vi "Ex2.vi"   [LabVIEW 2012]
uses:
  <userlib>/rosforlv/ROS/Code/SubVIs/BaxterSide.ctl
panel:
  # "Hit run to close and open the gripper"
types:
  T1 = typedef "BaxterSide.ctl" = enum16{"left", "right"}
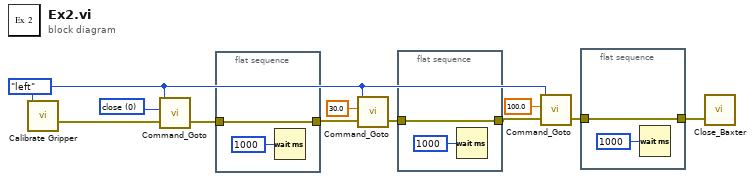
[diagram p0: block diagram]
diagram:
  w11 = u16 0 items=["close"=0, "open"=100] ("left gripper")
  w2 = BaxterSide."left" ("Side")
  n1 = call <userlib>:"Calibrate Gripper.vi"("Side"=w2) -> ("error out"=w10:errorcluster)  [unwired: 5 in]
  n2 = call <userlib>:"Command_Goto.vi"("Side"=w2, "Desired Position"=w11, "error in"=w10) -> ("error out"=w8:errorcluster)  [unwired: 3 in]
  n3 = flat-sequence {
    tunnel: [w12] -> w9
    tunnel: w8 -> [w12]
    frame #0 {
      n4 = Wait (ms)(milliseconds to wait=u32 1000) -> ()  [unwired: 1 out]
    }
  }
  n5 = call <userlib>:"Command_Goto.vi"("Side"=w2, "Desired Position"=sgl 30.0, "error in"=w9) -> ("error out"=w6:errorcluster)  [unwired: 3 in]
  n6 = flat-sequence {
    tunnel: [w14] -> w3
    tunnel: w6 -> [w14]
    frame #0 {
      n7 = Wait (ms)(milliseconds to wait=u32 1000) -> ()  [unwired: 1 out]
    }
  }
  n8 = call <userlib>:"Command_Goto.vi"("Side"=w2, "Desired Position"=sgl 100.0, "error in"=w3) -> ("error out"=w5:errorcluster)  [unwired: 3 in]
  n9 = flat-sequence {
    tunnel: [w16] -> w1
    tunnel: w5 -> [w16]
    frame #0 {
      n10 = Wait (ms)(milliseconds to wait=u32 1000) -> ()  [unwired: 1 out]
    }
  }
  n11 = call <userlib>:"Close_Baxter.vi"("error in"=w1) -> ()  [unwired: 3 in, 1 out]
